vi "Channel_Description_Global.vi"() -> ()   [LabVIEW 2021]
uses:
  ADAM Client/Sub VIs/ADAM Controls/Ch_description_ADAM.ctl
  ADAM Client/Sub VIs/ADAM Controls/Module_type_ADAM.ctl
  ADAM Client/Sub VIs/ADAM Controls/Function_ADAM.ctl
  ADAM Client/Sub VIs/ADAM Controls/Channel_State.ctl
  ADAM Client/Sub VIs/ADAM Controls/Calib_type_ADAM.ctl
  ADAM Client/Sub VIs/ADAM Controls/Address.ctl
panel:
  in  "Channel Description":T1[](array[typedef]) {"Duty" format="%016b"; "D" format="%#_5g"; "C" format="%#_5g"; "B" format="%#_5g"; "A" format="%#_5g"}
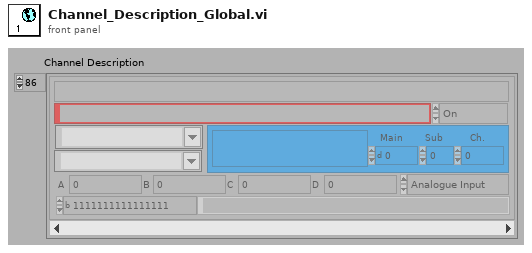
[diagram p1: front panel]
types:
  T1 = typedef "Ch_description_ADAM.ctl" = cluster{"Ch Name":string, "Type":T2, "Function":T3, "Ch State":T4, "Calibration type":T5, "A":dbl, "B":dbl, "C":dbl, "D":dbl, "Comments":string, "Address":T6, "String":string, "Duty":u16}
  T2 = typedef "Module_type_ADAM.ctl" = string
  T3 = typedef "Function_ADAM.ctl" = enum16{"Analogue Input", "Digital Input", "Event counter", "Event rate", "Analogue Output", "Digital Output", "Relay Output"}
  T4 = typedef "Channel_State.ctl" = enum16{"On", "Off", "Always On", "Always Off"}
  T5 = typedef "Calib_type_ADAM.ctl" = string
  T6 = typedef "Address.ctl" = cluster{"Main":i32, "Ch.":i32, "Sub":i32, "Port Name":string}
diagram:
